vi "UpdateStepScript.vi"(8 "error in (no error)":errorcluster, 11 "StepScript":T1[](array[typedef])) -> (0 "error out":errorcluster)   [LabVIEW 2016, in "SeqProcessor.lvlib"]
uses:
  SeqProcessor.lvlib
  controls/Step.ctl
  controls/StepType.ctl
  <vilib>/addons/PointValueMap/subVIs/Point_Write_variant.vi
  <vilib>/addons/PointValueMap/PointValueMap.lvlib
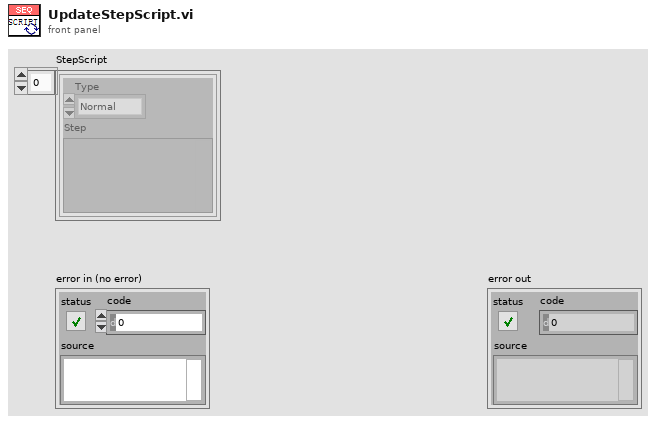
[diagram p1: front panel]
types:
  T1 = typedef "SeqProcessor.lvlib/Step.ctl" = cluster{"Type":T2, "Step":variant}
  T2 = typedef "SeqProcessor.lvlib/StepType.ctl" = enum16{"Normal", "Parallel", "Conditional", "Jump"}
  T3 = typedef "PointValueMap.lvlib/PointMap.ctl" = refnum<data-value>
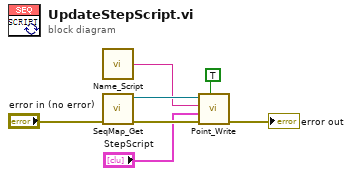
[diagram p0: block diagram]
diagram:
  n1 = call "Name_Script.vi"() -> ("StepScript"=w2:string)  [unwired: 5 in]
  n2 = call "SeqMap_Get.vi"("error in (no error)"="error in (no error)") -> ("error out"=w6:errorcluster, "SeqMap"=w5:T3)  [unwired: 9 in]
  n3 = call-poly <vilib>:"Point_Write.vi"("Auto Create?"=TRUE, "Error In"=w6, "Value"="StepScript", "Tag"=w2, "Map"=w5) -> ("Error Out"=→"error out":errorcluster)  [unwired: 5 in, 1 out]
